vi "ConvertSRs.vi"(11 "SRList":T1 {"SR#" format="%#_10g"}) -> (3 "SRlistString":string[][](array[string]))   [LabVIEW 2017, in "Client.lvlib" / "CommsServer.lvlib"]
uses:
  CommsServer.lvlib
  TypeDefs/SR List.ctl
  TypeDefs/SR Data.ctl
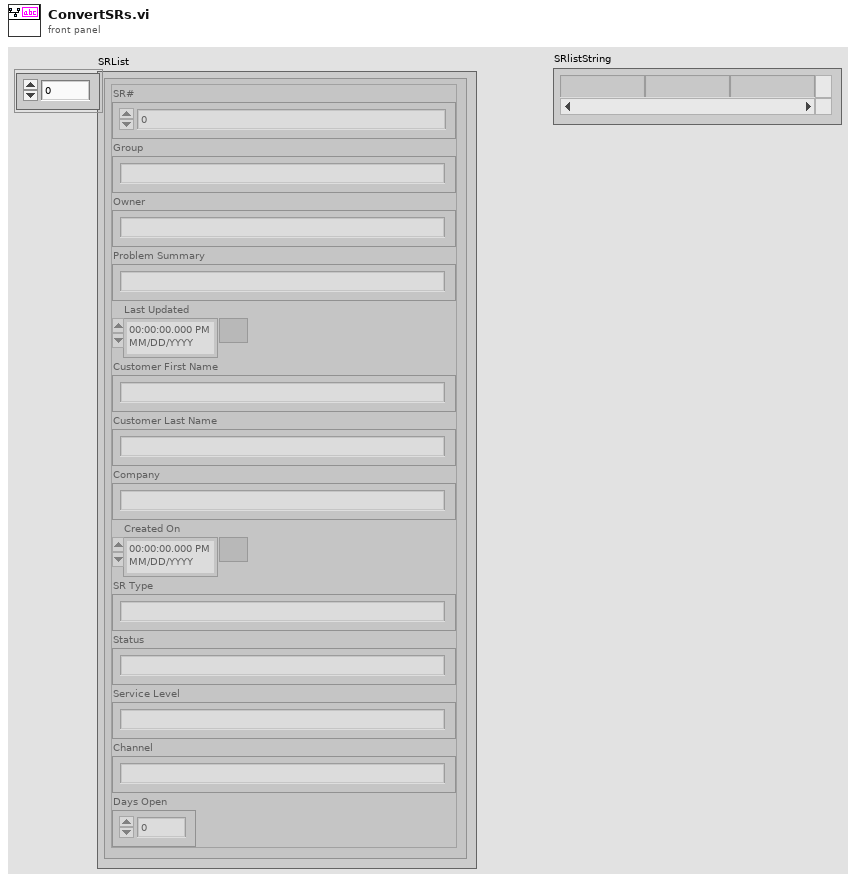
[diagram p1: front panel]
types:
  T1 = typedef "Client.lvlib/CommsServer.lvlib/SR List.ctl" = T2[]
  T2 = typedef "Client.lvlib/CommsServer.lvlib/SR Data.ctl" = cluster{"SR#":dbl, "Group":string, "Owner":string, "Problem Summary":string, "Last Updated":timestamp, "Customer First Name":string, "Customer Last Name":string, "Company":string, "Created On":timestamp, "SR Type":string, "Status":string, "Service Level":string, "Channel":string, "Days Open":dbl}
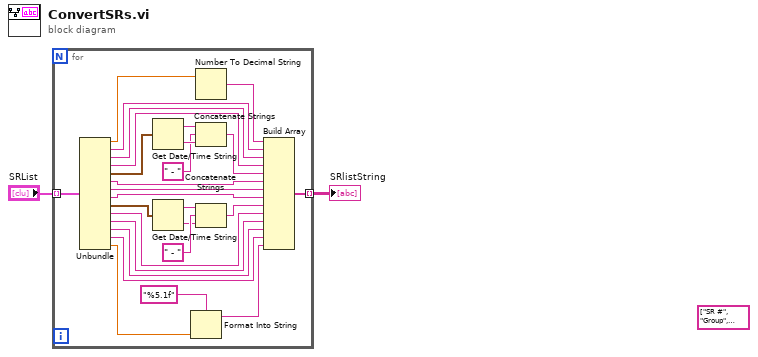
[diagram p0: block diagram]
diagram:
  (unwired) string[] ["SR #", "Group", "Owner", "Problem Summary", "Last Updated", "Customer First Name", "Customer Last Name", "Company", "Created On", "SR Type", "Status", "Service Level", "Channel", "Days Open"] ("Array")
  n1 = for {
    tunnel: "SRList" -> [w29] mode=indexing
    tunnel: [w4] -> w1 mode=indexing
    n2 = Unbundle(w29) -> ("SR#"=w28:dbl, "Group"=w26:string, "Owner"=w25:string, "Problem Summary"=w24:string, "Last Updated"=w23:timestamp, "Customer First Name"=w18:string, "Customer Last Name"=w17:string, "Company"=w16:string, "Created On"=w12:timestamp, "SR Type"=w10:string, "Status"=w9:string, "Service Level"=w8:string, "Channel"=w7:string, "Days Open"=w6:dbl)
    n3 = Get Date/Time String(seconds (now)=w23) -> (date string=w22:string, time string=w21:string)  [unwired: 2 in]
    n4 = Get Date/Time String(seconds (now)=w12) -> (date string=w13:string, time string=w14:string)  [unwired: 2 in]
    n5 = Format Into String(format string="%5.1f", w6) -> (resulting string=w5:string)  [unwired: 2 in, 1 out]
    n6 = Number To Decimal String(number=w28) -> (decimal integer string=w27:string)  [unwired: 1 in]
    n7 = Concatenate Strings(w22, " - " ("string"), w21) -> (w19:string)
    n8 = Concatenate Strings(w13, " - " ("string"), w14) -> (w11:string)
    n9 = Build Array(w27, w26, w25, w24, w19, w18, w17, w16, w11, w10, w9, w8, w7, w5) -> (w4:string[])
  }
  "SRlistString" <- w1
